vi "init.vi"(8 "error in (no error)":errorcluster, 11 "DataListenerThisComponent in":refnum<class "DataListenerThisComponent.lvclass">) -> (0 "error out":errorcluster, 3 "DataListenerThisComponent out":refnum<class "DataListenerThisComponent.lvclass">)   [LabVIEW 2012, in "DataListenerThisComponent.lvclass"]
doc: "Opens connections to the SubDataSVs. Assembles the URLs for the variables using information from the configuration and the variable names from the SubDataSV control linked to a typedef.\nThere is no need to update this VI; updating the typedef specifying the SubDataSVs is sufficient."
uses:
  DataListenerThisComponent.lvclass
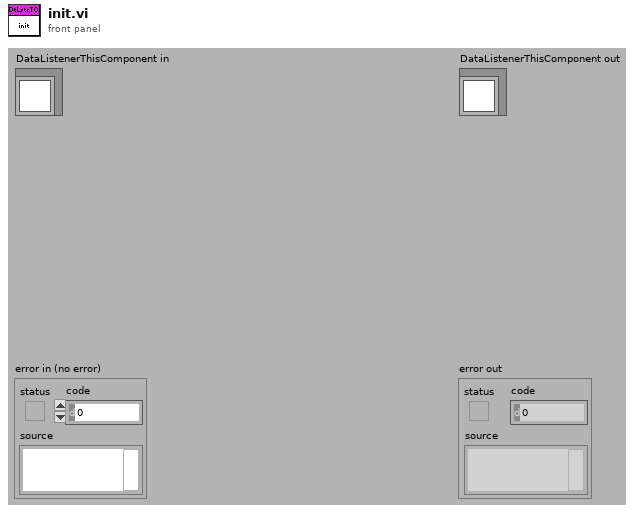
[diagram p1: front panel]
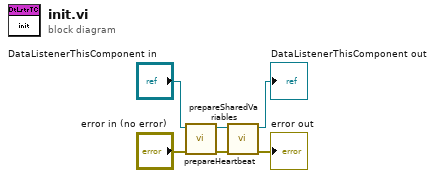
[diagram p0: block diagram]
diagram:
  n1 = call "prepareHeartbeat.vi"("error in (no error)"="error in (no error)", "DataListenerThisComponent in"="DataListenerThisComponent in") -> ("error out"=w2:errorcluster, "DataListenerThisComponent out"=w5:refnum<class "DataListenerThisComponent.lvclass">)  [unwired: 8 in]
  n2 = call "prepareSharedVariables.vi"("error in (no error)"=w2, "DataListenerThisComponent in"=w5) -> ("error out"=→"error out":errorcluster, "DataListenerThisComponent out"=→"DataListenerThisComponent out":refnum<class "DataListenerThisComponent.lvclass">)  [unwired: 8 in]
